vi "Image Path & Name Flir-Ax8.vi"(1 "Base Path":path) -> (0 "Appended Path":path)   [LabVIEW 2016]
panel:
  out "image name and formt output":string
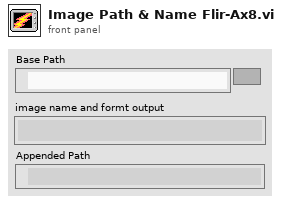
[diagram p1: front panel]
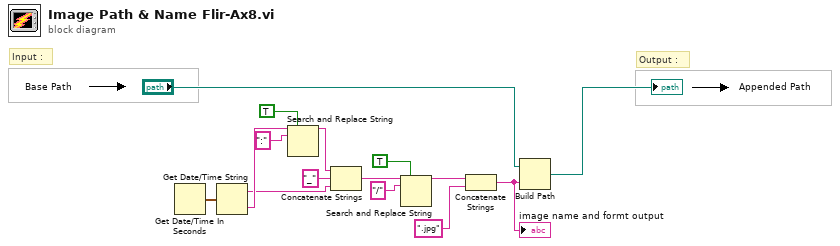
[diagram p0: block diagram]
diagram:
  # "Output :"
  # "Input :"
  n1 = Get Date/Time In Seconds() -> (seconds since 1Jan1904=w9:timestamp)
  n2 = Get Date/Time String(seconds (now)=w9) -> (date string=w4:string, time string=w6:string)  [unwired: 2 in]
  n3 = Search and Replace String(replace all?=TRUE ("replace all? (F)"), input string=w6, search string=":") -> (result string=w5:string)  [unwired: 5 in, 3 out]
  n4 = Concatenate Strings ("add")(w5, "_" ("string"), w4) -> (w3:string)
  n5 = Search and Replace String(replace all?=TRUE ("replace all? (F)"), input string=w3, search string="/") -> (result string=w2:string)  [unwired: 5 in, 3 out]
  n6 = Concatenate Strings ("add")(w2, ".jpg" ("string")) -> (w14:string)
  "image name and formt output" <- w14
  n7 = Build Path(base path="Base Path", name or relative path=w14) -> (appended path=→"Appended Path":path)
